vi "ReplicateFirstError.vi"(8 "error in (no error)":errorcluster, 11 "Sequence in":refnum<class "STEP.lvclass">[](array[class])) -> (0 "error out":errorcluster, 3 "Sequence out":refnum<class "STEP.lvclass">[](array[class]))   [LabVIEW 2014]
uses:
  Classes/STEP/STEP.lvclass
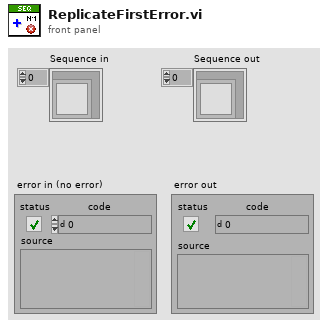
[diagram p1: front panel]
types:
  T1 = typedef "SeqLoop.lvlib/LogicParsedExpression.ctl" = cluster{"RPN ":string[], "Variables":string[], "Ctes":string[], "Formula":string, "Message":string}
  T2 = typedef "Seq-MathLoop.lvlib/LogicParsedExpression.ctl" = cluster{"RPN ":string[], "Variables":string[], "Ctes":string[], "Formula":string, "Message":string}
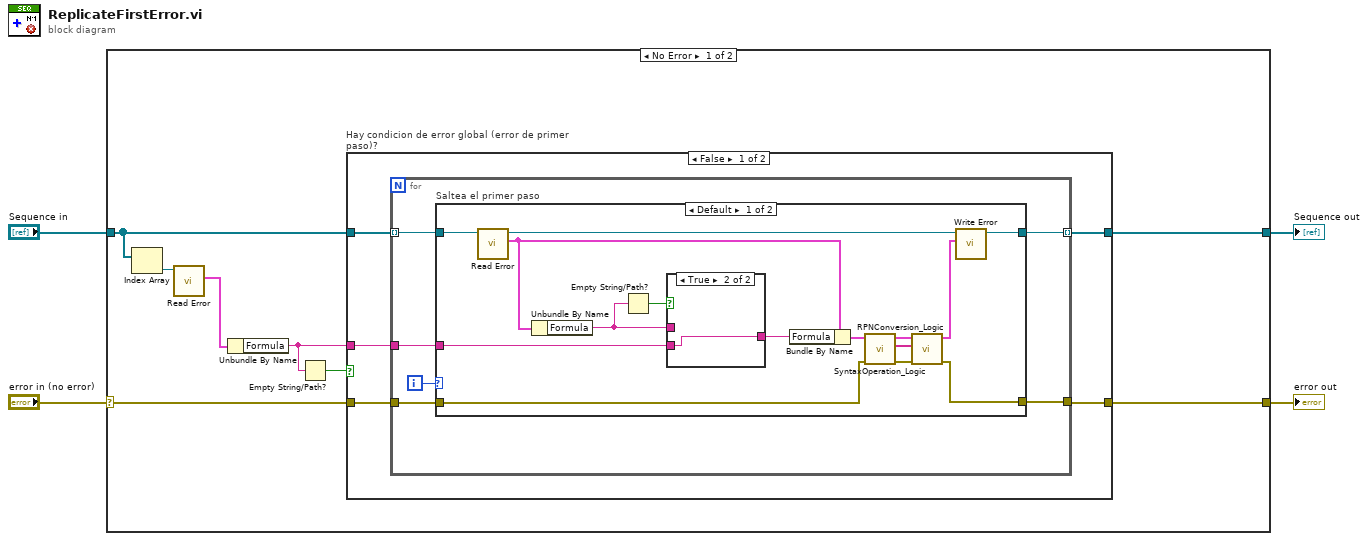
[diagram p0: block diagram]
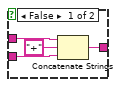
[diagram p2: hidden frame]
diagram:
  n1 = case shown="No Error" "error in (no error)" {
    selector: "error in (no error)" -> [w11 w49]
    tunnel: [w12 w49] -> w4
    tunnel: "Sequence in" -> [w6 w48]
    tunnel: [w5 w48] -> w1
    frame No Error {
      n2 = Index Array(array=w6) -> (element=w10:refnum<class "STEP.lvclass">)  [unwired: 1 in]
      n3 = call "Read Error .vi"("STEP in"=w10) -> ("Error"=w9:T1)  [unwired: 9 in, 1 out]
      n4 = Unbundle By Name(w9) -> ("Formula"=w8:string)
      n5 = Empty String/Path?(string/path=w8) -> (empty?=w7:bool)
      n6 = case "Hay condicion de error global (error de primer paso)?" shown="False" w7 {
        tunnel: w6 -> [w17 w47]
        tunnel: [w16 w47] -> w5
        tunnel: [w15 w46] -> w12
        tunnel: w11 -> [w14 w46]
        tunnel: w8 -> [w13 _]
        frame False {
          n7 = for {
            tunnel: w17 -> [w23] mode=indexing
            tunnel: w13 -> [w21]
            tunnel: [w22] -> w16 mode=indexing
            tunnel: w14 -> [w20]
            tunnel: [w19] -> w15
            i -> [w18]
            n8 = case "Saltea el primer paso" shown="Default" w18 {
              tunnel: w23 -> [w38 w45]
              tunnel: [w37 w45] -> w22
              tunnel: w21 -> [w36 _]
              tunnel: w20 -> [w35 w44]
              tunnel: [w34 w44] -> w19
              frame Default {
                n9 = call "Read Error .vi"("STEP in"=w38) -> ("Error"=w25:T1, "STEP out"=w26:refnum<class "STEP.lvclass">)  [unwired: 9 in]
                n10 = Unbundle By Name(w25) -> ("Formula"=w32:string)
                n11 = Empty String/Path?(string/path=w32) -> (empty?=w33:bool)
                n12 = case shown="True" w33 {
                  tunnel: w32 -> [w42 _]
                  tunnel: w36 -> [w41 w43]
                  tunnel: [w39 w43] -> w27
                  frame False {
                    n13 = Concatenate Strings(w42, "+" ("string"), w41) -> (w39:string)
                  }
                  frame True {
                  }
                }
                n14 = Bundle By Name(cluster=w25, "Formula"=w27) -> (w28:T1)
                n15 = call "SyntaxOperation_Logic.vi"("error in (no error)"=w35, "Logical Parsed Expression"=w28) -> ("error out"=w29:errorcluster, "Token"=w30:string[], "Logical Parsed Expression Out"=w31:T2)  [unwired: 6 in, 1 out]
                n16 = call "RPNConversion_Logic.vi"("error in"=w29, "Token"=w30, "Logical Parsed Expression"=w31) -> ("error out"=w34:errorcluster, "Logical Parsed Expression Out"=w24:T2)  [unwired: 7 in]
                n17 = call "Write Error .vi"("Error"=w24, "STEP in"=w26) -> ("STEP out"=w37:refnum<class "STEP.lvclass">)  [unwired: 9 in]
              }
              frame 0 {
              }
            }
          }
        }
        frame True {
        }
      }
    }
    frame Error {
    }
  }
  "error out" <- w4
  "Sequence out" <- w1
